vi "ziSetValueBinaryArray.vi"(3 "Error In":errorcluster, 4 "Values":string[](array[string]), 5 "Paths":string[](array[string]), 6 "Handle In":T1 {"Handle" format="0x%08x"; "Conn" format="0x%08x"}) -> (0 "Error Out":errorcluster, 2 "Handle Out":T1 {"Handle" format="0x%08x"; "Conn" format="0x%08x"})   [LabVIEW 2016, in "Zurich Instruments LabOne.lvlib"]
doc: "This vi sets values to the nodes specified in Path to Value. More than one node can be set if a wildcard is used in Path. The i-th element of Paths receives the i-th value of Values."
uses:
  Zurich Instruments LabOne.lvlib
  ziTypeHandle.ctl
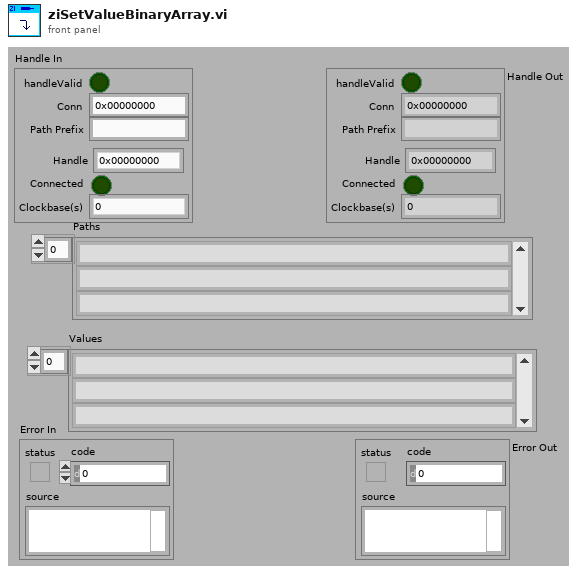
[diagram p1: front panel]
types:
  T1 = typedef "Zurich Instruments LabOne.lvlib/ziTypeHandle.ctl" = cluster{"handleValid":bool, "Conn":u64, "Path Prefix":string, "Handle":u64, "Connected":bool, "Clockbase(s)":dbl}
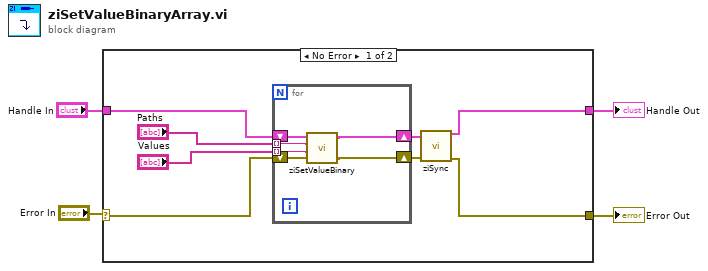
[diagram p0: block diagram]
diagram:
  n1 = case shown="No Error" "Error In" {
    selector: "Error In" -> [w10 w20]
    tunnel: [w6 w20] -> w4
    tunnel: [w5 w19] -> w3
    tunnel: "Handle In" -> [w9 w19]
    frame No Error {
      n2 = for {
        tunnel: "Paths" -> [w13] mode=indexing
        tunnel: "Values" -> [w14] mode=indexing
        shift-right: [w16] -> w7
        shift-left: w10 -> [w15]
        shift-right: [w17] -> w8
        shift-left: w9 -> [w18]
        n3 = call "ziSetValueBinary.vi"("Error In"=w15, "Data"=w14, "Path"=w13, "Handle In"=w18) -> ("Error Out"=w16:errorcluster, "Handle Out"=w17:T1)  [unwired: 1 in]
      }
      n4 = call "ziSync.vi"("Handle In"=w8, "Error In"=w7) -> ("Handle Out"=w5:T1, "Error Out"=w6:errorcluster)  [unwired: 12 in]
    }
    frame Error {
    }
  }
  "Error Out" <- w4
  "Handle Out" <- w3
